vi "Optimizer.vi"(11 "Optimize Parameters":T1={"Volt Step"={"X"=0.01, "Y"=0.01, "Z"=0.0}, "Num Iterations"=1, "Dwell Time (ms)"=100, "Volts Range"={"X"=0.1, "Y"=0.1, "Z"=0.0}, "Method"={"X"=enum."Max", "Y"=enum."Max", "Z"=enum."Max"}} {"Volts Range"."Z" min=0.0; "Volts Range"."Y" min=0.0; "Volts Range"."X" min=0.0; "Dwell Time (ms)" min=0; "Num Iterations" min=1 step=1; "Volt Step"."Z" min=0.0; "Volt Step"."Y" min=1e-06; "Volt Step"."X" min=1e-06}) -> ()   [LabVIEW 2012]
uses:
  Strict Type Def - Optimize Parameters Cluster.ctl
  Channels.vi
  Global Vars.vi
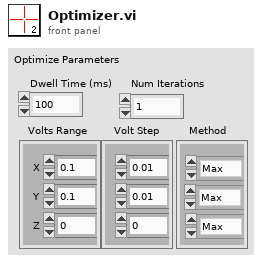
[diagram p1: front panel]
types:
  T1 = typedef "Strict Type Def - Optimize Parameters Cluster.ctl" = cluster{"Volt Step":cluster{"X":dbl, "Y":dbl, "Z":dbl}, "Num Iterations":i32, "Dwell Time (ms)":i32, "Volts Range":cluster{"X":dbl, "Y":dbl, "Z":dbl}, "Method":cluster{"X":enum16{"Max", "Gaussian"}, "Y":enum16{"Max", "Gaussian"}, "Z":enum16{"Max", "Gaussian"}}}
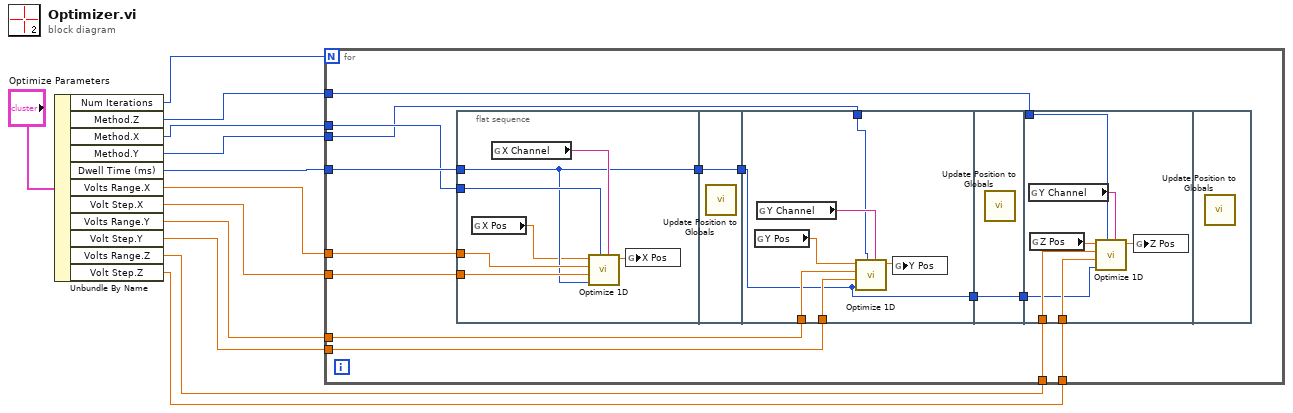
[diagram p0: block diagram]
diagram:
  n1 = Unbundle By Name("Optimize Parameters") -> ("Num Iterations"=w5:i32, "Method.Z"=w1:enum16{"Max", "Gaussian"}, "Method.X"=w2:enum16{"Max", "Gaussian"}, "Method.Y"=w10:enum16{"Max", "Gaussian"}, "Dwell Time (ms)"=w12:i32, "Volts Range.X"=w9:dbl, "Volt Step.X"=w8:dbl, "Volts Range.Y"=w7:dbl, "Volt Step.Y"=w6:dbl, "Volts Range.Z"=w4:dbl, "Volt Step.Z"=w3:dbl)
  n2 = for {
    N: w5 -> [_]
    tunnel: w12 -> [w26]
    tunnel: w2 -> [w23]
    tunnel: w10 -> [w22]
    tunnel: w9 -> [w21]
    tunnel: w8 -> [w20]
    tunnel: w7 -> [w19]
    tunnel: w6 -> [w18]
    tunnel: w4 -> [w17]
    tunnel: w3 -> [w16]
    tunnel: w1 -> [w13]
    n3 = flat-sequence {
      tunnel: w26 -> [w28]
      tunnel: [w28] -> w25
      tunnel: w23 -> [w31]
      tunnel: w21 -> [w30]
      tunnel: w20 -> [w29]
      tunnel: w25 -> [w34]
      tunnel: [w34] -> w24
      tunnel: w24 -> [w35]
      tunnel: w22 -> [w39]
      tunnel: w19 -> [w37]
      tunnel: w18 -> [w36]
      tunnel: [w35] -> w14
      tunnel: [w42] -> w15
      tunnel: w14 -> [w42]
      tunnel: w17 -> [w47]
      tunnel: w16 -> [w46]
      tunnel: w15 -> [w45]
      tunnel: w13 -> [w44]
      frame #0 {
        n4 = global read "Global Vars.vi" "X Pos"() -> (w27:dbl)
        n5 = global read "Channels.vi" "X Channel"() -> (w32:tag)
        n6 = call "Optimize 1D.vi"("AO Channel"=w32, "Fit Method"=w31, "Dwell Time (ms)"=w28, "Volt Step"=w29, "Volt Range"=w30, "Curr Pos"=w27) -> ("Final Pos"=w33:dbl)  [unwired: 5 in]
        n7 = global write "Global Vars.vi" "X Pos"(w33) -> ()
      }
      frame #1 {
        n8 = call "Update Position to Globals.vi"() -> ()  [unwired: 11 in, 1 out]
      }
      frame #2 {
        n9 = global read "Global Vars.vi" "Y Pos"() -> (w38:dbl)
        n10 = global read "Channels.vi" "Y Channel"() -> (w41:tag)
        n11 = call "Optimize 1D.vi"("AO Channel"=w41, "Fit Method"=w39, "Dwell Time (ms)"=w35, "Volt Step"=w36, "Volt Range"=w37, "Curr Pos"=w38) -> ("Final Pos"=w40:dbl)  [unwired: 5 in]
        n12 = global write "Global Vars.vi" "Y Pos"(w40) -> ()
      }
      frame #3 {
        n13 = call "Update Position to Globals.vi"() -> ()  [unwired: 11 in, 1 out]
      }
      frame #4 {
        n14 = global read "Channels.vi" "Y Channel"() -> (w49:tag)
        n15 = global read "Global Vars.vi" "Z Pos"() -> (w48:dbl)
        n16 = call "Optimize 1D.vi"("AO Channel"=w49, "Fit Method"=w44, "Dwell Time (ms)"=w45, "Volt Step"=w46, "Volt Range"=w47, "Curr Pos"=w48) -> ("Final Pos"=w43:dbl)  [unwired: 5 in]
        n17 = global write "Global Vars.vi" "Z Pos"(w43) -> ()
      }
      frame #5 {
        n18 = call "Update Position to Globals.vi"() -> ()  [unwired: 11 in, 1 out]
      }
    }
  }
